vi "Host - Auxillary BMS Data (SubVI).vi"(11 "Aux BMS Data":string) -> (1 "Pack SOC":dbl, 2 "Load Current":dbl, 3 "Pack Voltage":dbl, 4 "Temp":dbl)   [LabVIEW 2021]
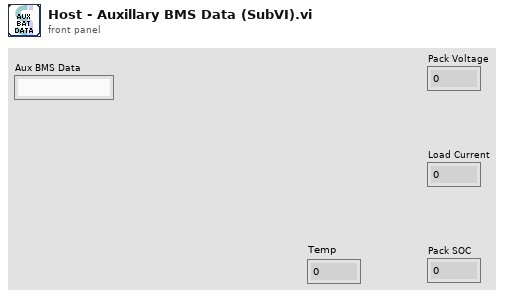
[diagram p1: front panel]
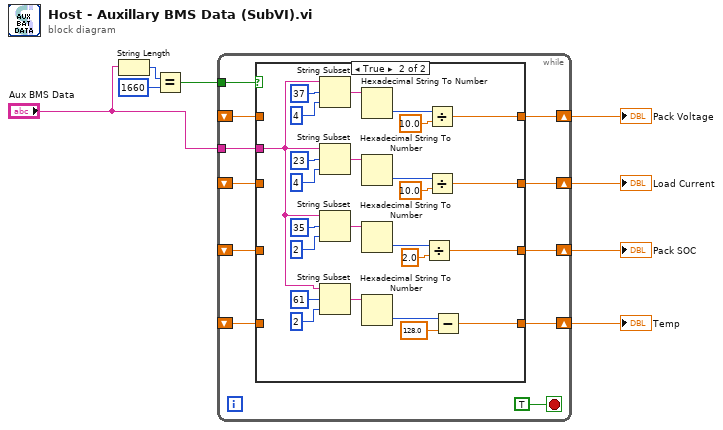
[diagram p0: block diagram]
diagram:
  n1 = String Length(string="Aux BMS Data") -> (length=w3:i32)
  n2 = Equal?(x=w3, y=1660) -> (x = y?=w2:bool)
  n3 = while {
    tunnel: "Aux BMS Data" -> [w16]
    shift-right: [w18] -> w7
    shift-left: _ -> [w11]
    shift-right: [w19] -> w8
    shift-left: _ -> [w12]
    shift-right: [w17] -> w6
    shift-left: _ -> [w13]
    tunnel: w2 -> [w14]
    shift-right: [w10] -> w1
    shift-left: _ -> [w9]
    stop <- TRUE stop-if-true
    n4 = case shown="True" w14 {
      tunnel: [w22 w48] -> w19
      tunnel: [w21 w47] -> w18
      tunnel: [w23 w46] -> w17
      tunnel: w16 -> [_ w25]
      tunnel: w13 -> [w23 _]
      tunnel: w12 -> [w22 _]
      tunnel: w11 -> [w21 _]
      tunnel: [w20 w24] -> w10
      tunnel: w9 -> [w20 _]
      frame False {
      }
      frame True {
        n5 = String Subset(string=w25, offset (0)=37, length (rest)=4 ("length (rest)")) -> (substring=w39:string)
        n6 = String Subset(string=w25, offset (0)=23, length (rest)=4 ("length (rest)")) -> (substring=w37:string)
        n7 = String Subset(string=w25, offset (0)=35, length (rest)=2 ("length (rest)")) -> (substring=w38:string)
        n8 = String Subset(string=w25, offset (0)=61, length (rest)=2 ("length (rest)")) -> (substring=w30:string)
        n9 = Hexadecimal String To Number(string=w39) -> (number=w45:u32)  [unwired: 2 in, 1 out]
        n10 = Hexadecimal String To Number(string=w37) -> (number=w41:u32)  [unwired: 2 in, 1 out]
        n11 = Hexadecimal String To Number(string=w38) -> (number=w43:u32)  [unwired: 2 in, 1 out]
        n12 = Hexadecimal String To Number(string=w30) -> (number=w29:u32)  [unwired: 2 in, 1 out]
        n13 = Divide(x=w43, y=2.0) -> (x/y=w47:dbl)
        n14 = Divide(x=w45, y=10.0) -> (x/y=w46:dbl)
        n15 = Divide(x=w41, y=10.0) -> (x/y=w48:dbl)
        n16 = Subtract(x=w29, y=128.0) -> (x-y=w24:dbl)
      }
    }
  }
  "Load Current" <- w8
  "Pack SOC" <- w7
  "Pack Voltage" <- w6
  "Temp" <- w1
